vi "数据库查询.vi"() -> ()   [LabVIEW 2018]
uses:
  NPOI/net40/yt_ExcelLibrary.dll
  <vilib>/addons/database/Connection.llb/DB Tools Open Connec (String).vi
  <vilib>/addons/database/NI_Database_API.lvlib
  <vilib>/Utility/NIReport.llb/NI_report.lvclass
  <vilib>/addons/_office/NI_ReportGenerationToolkit.lvlib
  <vilib>/Utility/NIReport.llb/Excel/NI_Excel.lvclass
  <vilib>/addons/_office/_exclsub.llb/font.ctl
  <vilib>/ptbypt/NI_PtbyPt.lvlib
  FreeMem.dll
  <vilib>/addons/_office/excel.llb/Excel Easy Table (str).vi
panel:
  out "错误输出":errorcluster
  out "数字(0-1)":dbl
  out "Elapsed Time (s)":dbl caption="已用时间(s)"
  out "2天时间到释放资源":bool caption="结束"
  in  "Main Tab":enum32{""}(tab)
  in  "查询结果":i32(listbox)
  in  "时间范围OFF":bool
  out "查询状态":string
  in  "总成码OFF":bool
  in  "总成码":string
  in  "导出":bool
  in  "退出":bool
  in  "查询":bool
  in  "另存为":bool
  in  "二维码OFF":bool
  in  "二维码":string
  in  "结束日期":timestamp
  in  "起始日期":timestamp
  in  "数据类型":u16(ring) items=["ALL", "Online", "Offline", "Rework", "70站"]
  in  "产品状态":u16(ring) items=["ALL", "OK", "NG"]
  # "历史数据查询"
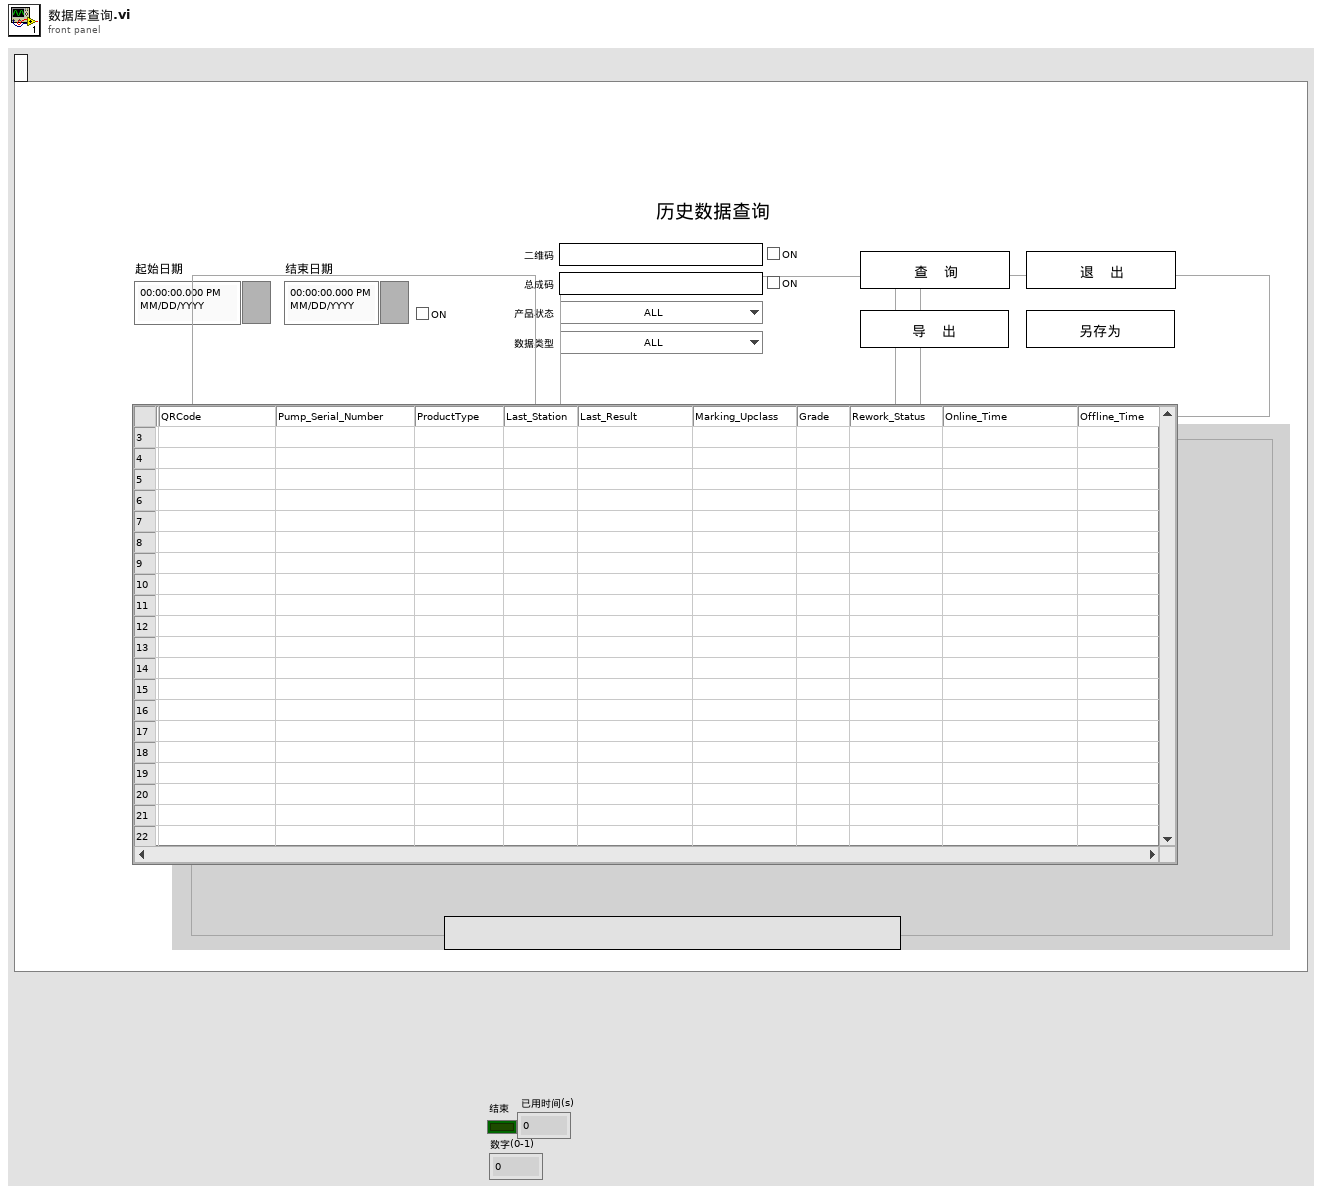
[diagram p1: front panel]
types:
  T1 = typedef "NI_ReportGenerationToolkit.lvlib/font.ctl" = cluster{"font name":string, "font size":dbl, "bold":u16, "italic":u16, "underline":u16, "strike through":u16, "font color":u32}
  T2 = enum16{"Standard Report", "HTML", "Word", "Excel"}
  T3 = enum16{"maximized", "minimized", "normal", "no change"}
  T4 = enum32{"Invalid", "Standard", "Closed", "Hidden", "Minimized", "Maximized"}
  T5 = typedef "NI_Database_API.lvlib/Conn ObjectReference.ctl" = refnum<k1>
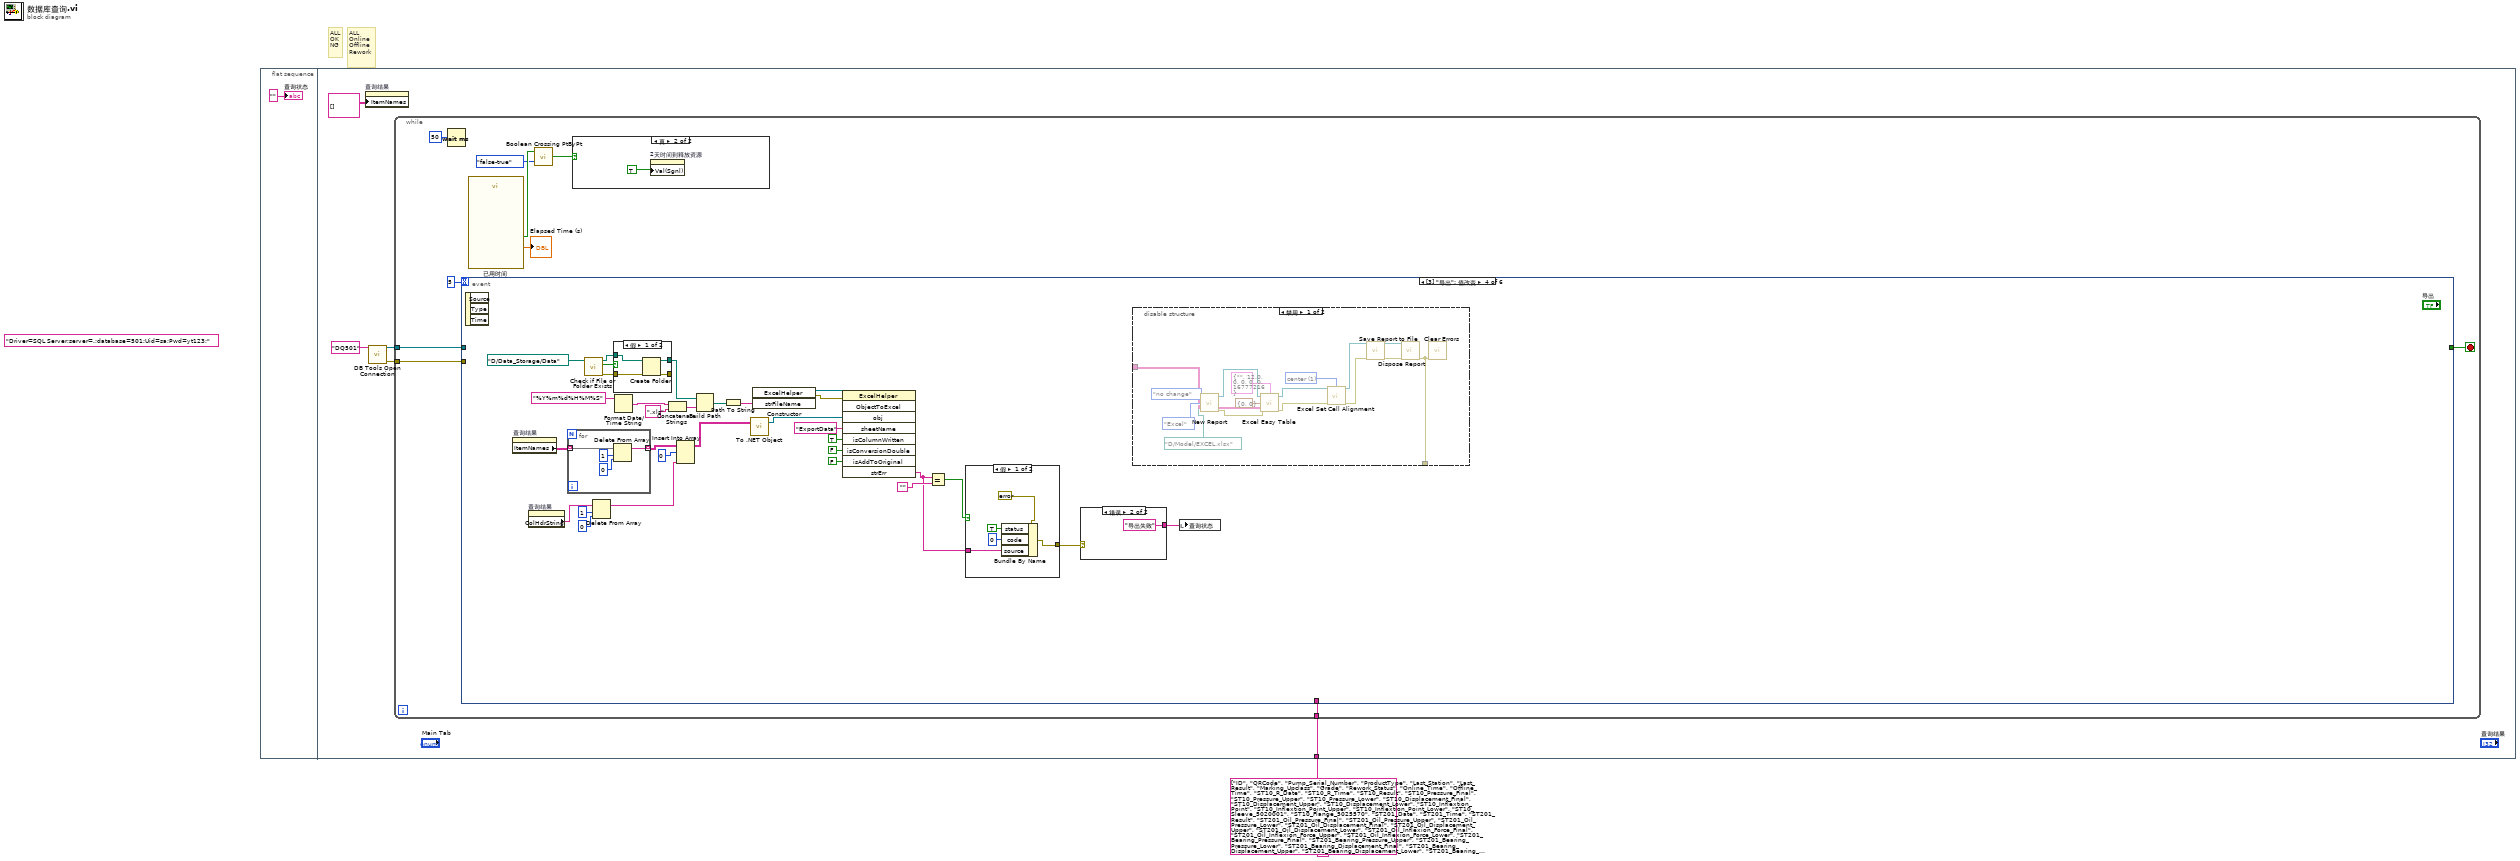
[diagram p0: block diagram]
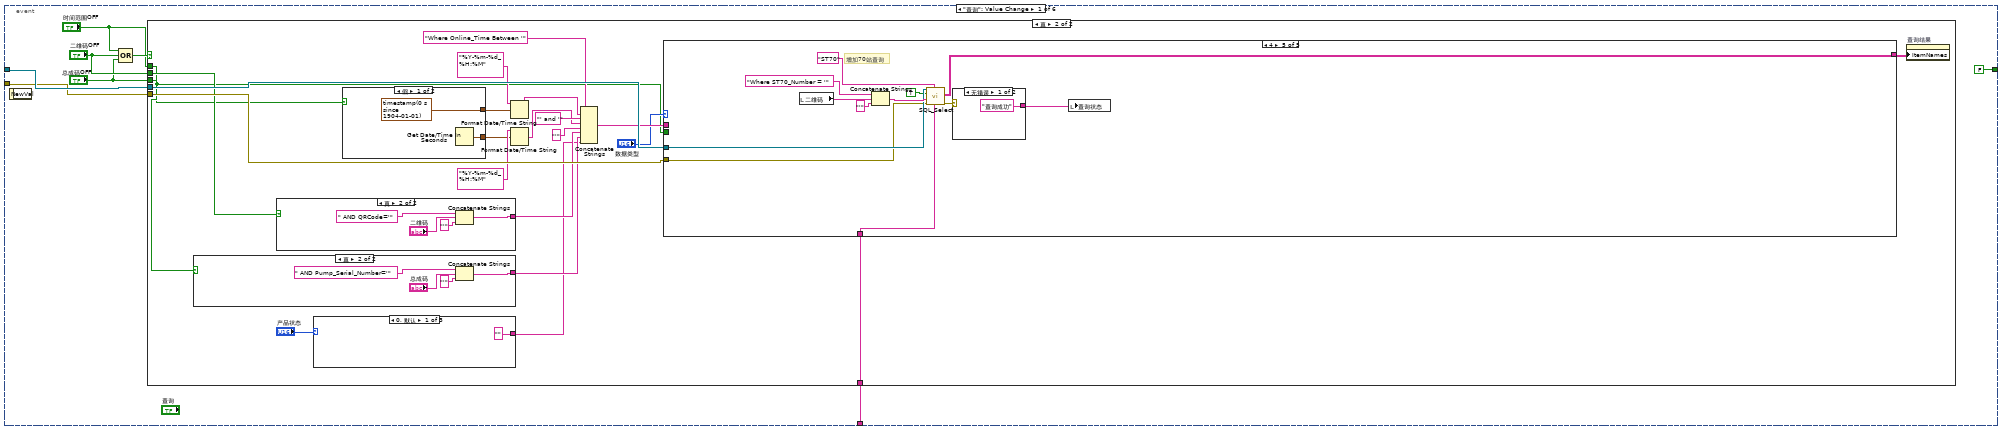
[diagram p3: hidden frame]
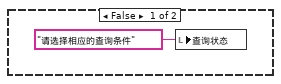
[diagram p4: hidden frame]
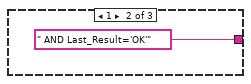
[diagram p5: hidden frame]
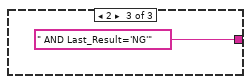
[diagram p6: hidden frame]
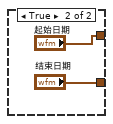
[diagram p7: hidden frame]
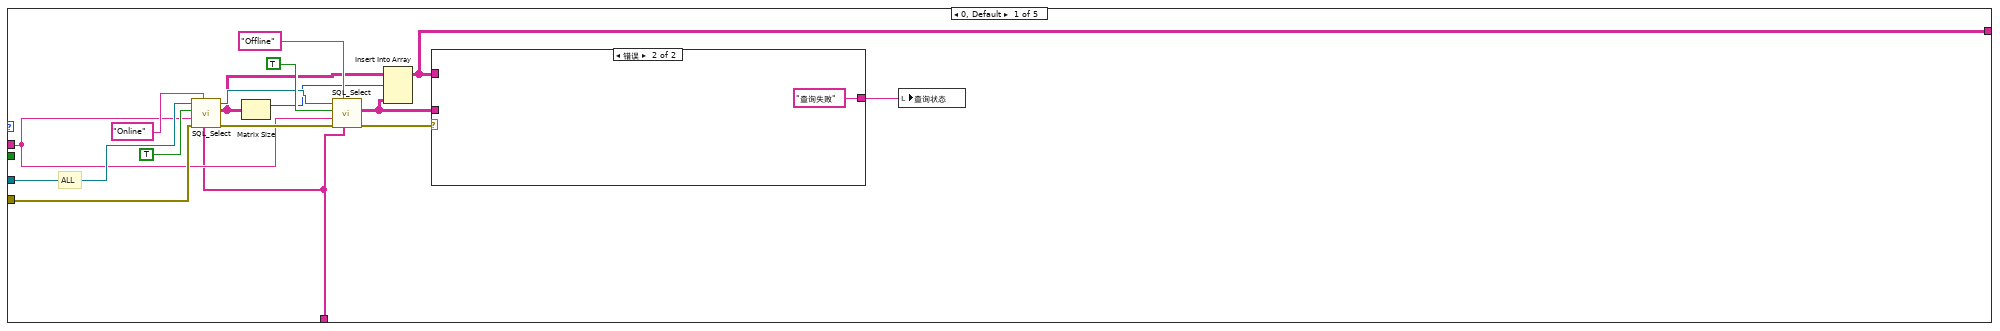
[diagram p8: hidden frame]
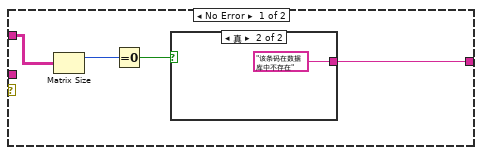
[diagram p9: hidden frame]
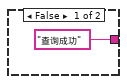
[diagram p10: hidden frame]
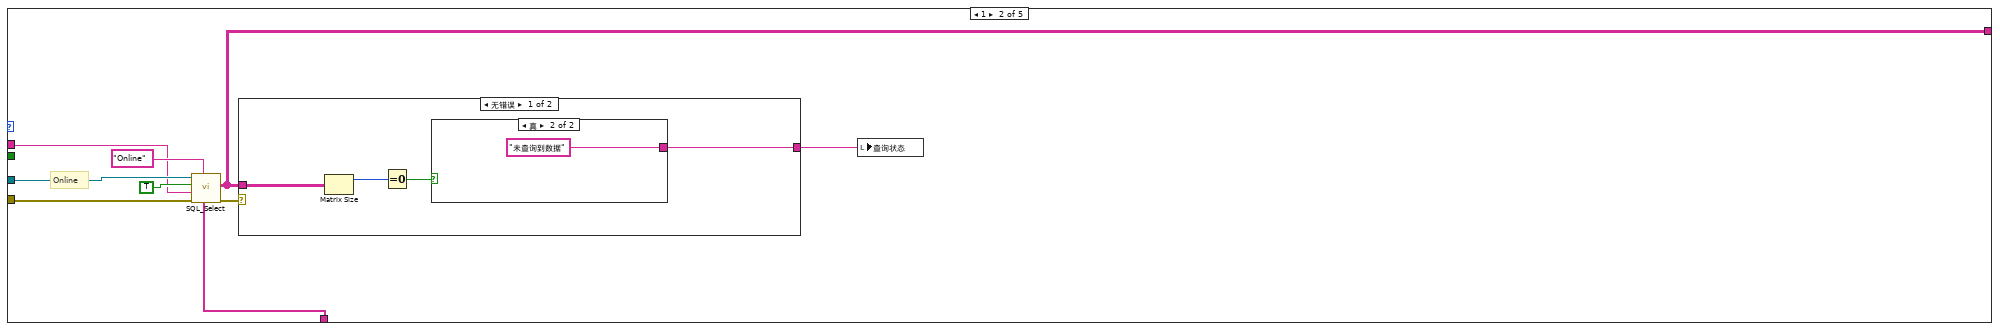
[diagram p11: hidden frame]
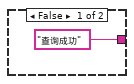
[diagram p12: hidden frame]
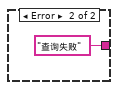
[diagram p13: hidden frame]
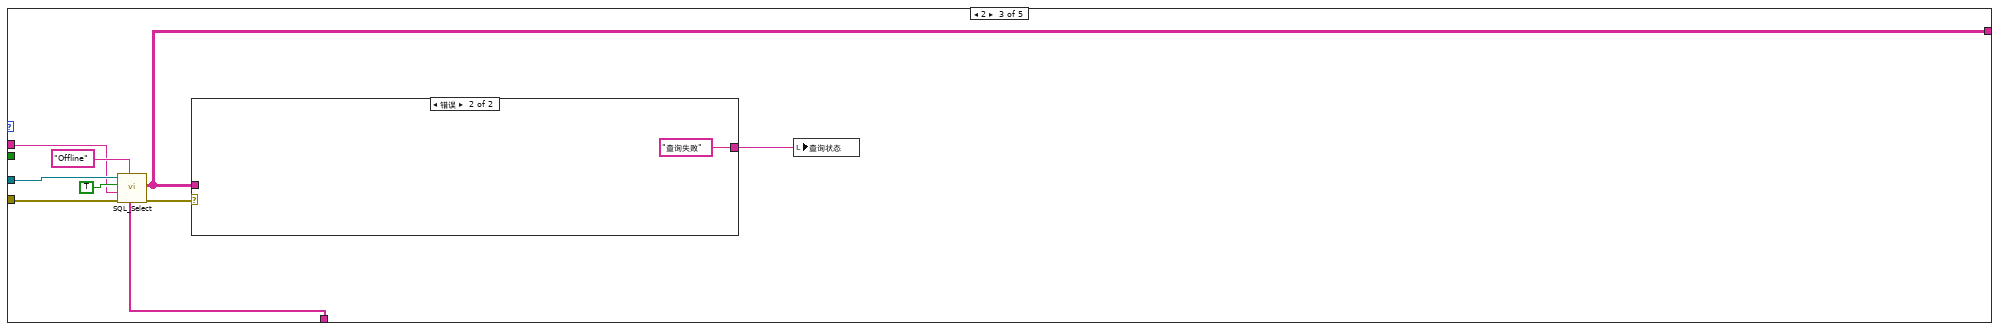
[diagram p14: hidden frame]
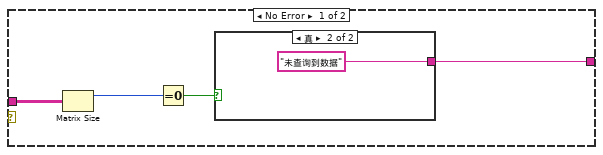
[diagram p15: hidden frame]
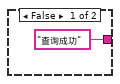
[diagram p16: hidden frame]
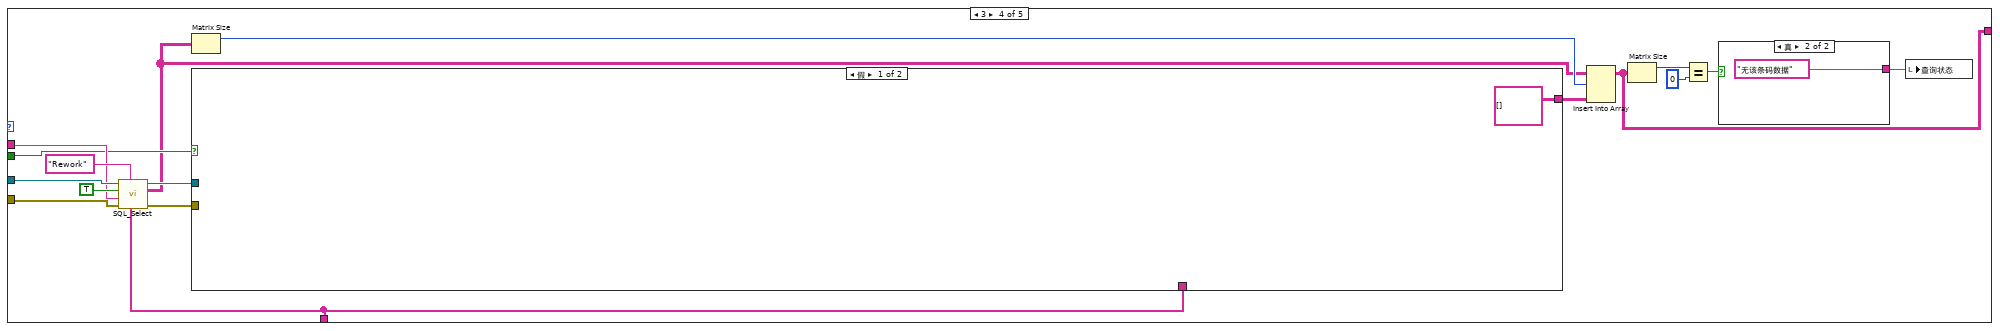
[diagram p17: hidden frame]
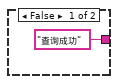
[diagram p18: hidden frame]
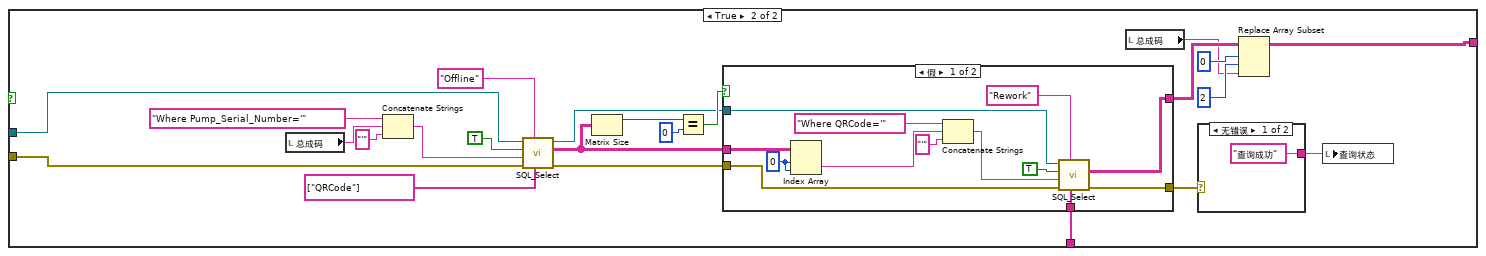
[diagram p19: hidden frame]
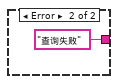
[diagram p20: hidden frame]
diagram:
  (unwired) "Driver=SQL Server;server=.;database=501;Uid=sa;Pwd=yt123;"
  # "ALL\nOK\nNG"
  # "ALL\nOnline\nOffline\nRework"
  n1 = flat-sequence {
    tunnel: string[] ["ID", "QRCode", "Pump_Serial_Number", "ProductType", "Last_Station", "Last_Result", "Marking_Upclass", "Grade", "Rework_Status", "Online_Time", "Offline_Time", "ST10_R_Date", "ST10_R_Time", "ST10_Result", "ST10_Pressure_Final", "ST10_Pressure_Upper", "ST10_Pressure_Lower", "ST10_Displacement_Final", "ST10_Displacement_Upper", "ST10_Displacement_Lower", "ST10_Inflextion_Point", "ST10_Inflextion_Point_Upper", "ST10_Inflextion_Point_Lower", "ST10_Sleeve_5020001", "ST10_Flange_5025570", "ST201_Date", "ST201_Time", "ST201_Result", "ST201_Oil_Pressure_Final", "ST201_Oil_Pressure_Upper", "ST201_Oil_Pressure_Lower", "ST201_Oil_Displacement_Final", "ST201_Oil_Displacement_Upper", "ST201_Oil_Displacement_Lower", "ST201_Oil_Inflexion_Force_Final", "ST201_Oil_Inflexion_Force_Upper", "ST201_Oil_Inflexion_Force_Lower", "ST201_Bearing_Pressure_Final", "ST201_Bearing_Pressure_Upper", "ST201_Bearing_Pressure_Lower", "ST201_Bearing_Displacement_Final", "ST201_Bearing_Displacement_Upper", "ST201_Bearing_Displacement_Lower", "ST201_Bearing_Inflexion_Force_Final", "ST201_Bearing_Inflexion_Force_Upper", "ST201_Bearing_Inflexion_Force_Lower", "ST202_Date", "ST202_Time", "ST202_Result", "ST202_Pressure_Final", "ST202_Pressure_Upper", "ST202_Pressure_Lower", "ST202_Displacement_Final", "ST202_Displacement_Upper", "ST202_Displacement_Lower", "ST202_Sealing_5026269", "ST202_Flange_5025570", "ST202_Shaft_5020526", "ST202_Ring_5020571", "ST202_Needle_bearing_5020570", "ST301_Date", "ST301_Time", "ST301_Result", "ST301_Shield", "ST301_Magnetic_flux_Left", "ST301_Magnetic_flux_Right", "ST301_Magnetic_flux_Upper", "ST301_Magnetic_flux_Lower", "ST301_PanelNumber", "ST302_Date", "ST302_Time", "ST302_Result", "ST302_PanelNumber", "ST303_Date", "ST303_Time", "ST303_Result", "ST303_PanelNumber", "ST303_Cam_ring_5020689", "ST303_Pin_5026280", "ST303_Rotor_5018111", "ST401_Date", "ST401_Time", "ST401_Result", "ST401_Shield", "ST401_PanelNumber", "ST402_Date", "ST402_Time", "ST402_Result", "ST402_Shield", "ST402_PanelNumber", "ST501_Date", "ST501_Time", "ST501_Result", "ST501_Shield", "ST501_PanelNumber", "ST502_Date", "ST502_Time", "ST502_Result", "ST502_PanelNumber", "ST502_Pressure_Final1", "ST502_Pressure_Upper1", "ST502_Pressure_Lower1", "ST502_Distance_Final1", "ST502_Distance_Upper1", "ST502_Distance_Lower1", "ST502_Pressure_Final2", "ST502_Pressure_Upper2", "ST502_Pressure_Lower2", "ST502_Distance_Final2", "ST502_Distance_Upper2", "ST502_Distance_Lower2", "ST502_Inflexion_force_Left_Final", "ST502_Inflexion_force_Left_Upper", "ST502_Inflexion_force_Left_Lower", "ST502_Inflexion_force_Right_Final", "ST502_Inflexion_force_Right_Upper", "ST502_Inflexion_force_Right_Lower", "ST503_Date", "ST503_Time", "ST503_Result", "ST503_PanelNumber", "ST503_Pin", "ST503_Position_degree", "ST504_Date", "ST504_Time", "ST504_Result", "ST504_PanelNumber", "ST504_Small_Sealing_Ring_Exit", "ST504_Small_Sealing_Ring_Excess", "ST504_Big_Sealing_Ring_Exit", "ST504_Big_Sealing_Ring_Number", "ST504_Retaining_Ring_LH2110811", "ST504_Pressure_Plate_5020472", "ST504_O_ring_5003059", "ST504_O_ring_5003061", "ST504_Spring_Dowel_Pin_5018182", "ST601_Date", "ST601_Time", "ST601_Result", "ST601_PanelNumber", "ST602_Date", "ST602_Time", "ST602_Result", "ST602_PanelNumber", "ST603_Date", "ST603_Time", "ST603_Result", "ST603_PanelNumber", "ST603_Spring_Retainer_5020834", "ST603_Spring_5024602", "ST603_Retaining_ring_5018568", "ST603_Disc_spring_5005082", "ST603_Bushing_5024673", "ST70_Number", "ST70_Date", "ST70_Time", "ST70_Result", "ST70_Pressure_Final1", "ST70_Pressure_Upper1", "ST70_Pressure_Lower1", "ST70_Distance_Final1", "ST70_Distance_Upper1", "ST70_Distance_Lower1", "ST70_Pressure_Final2", "ST70_Pressure_Upper2", "ST70_Pressure_Lower2", "ST70_Distance_Final2", "ST70_Distance_Upper2", "ST70_Distance_Lower2", "ST70_Inflexion_force_Left_Final", "ST70_Inflexion_force_Left_Upper", "ST70_Inflexion_force_Left_Lower", "ST70_Inflexion_force_Right_Final", "ST70_Inflexion_force_Right_Upper", "ST70_Inflexion_force_Right_Lower", "ST70_Housing_5025351", "ST70_Bushing_5025400", "ST80_Date", "ST80_Time", "ST80_Result", "ST80_Flat_Sael_5020064", "ST80_Spring_5024883", "ST80_Spring_Plate_5025473", "ST901_Date", "ST901_Time", "ST901_Result", "ST901_Torque1", "ST901_Angle1", "ST901_Gradient1", "ST901_Torque2", "ST901_Angle2", "ST901_Gradient2", "ST901_Torque3", "ST901_Angle3", "ST901_Gradient3", "ST901_Torque4", "ST901_Angle4", "ST901_Gradient4", "ST901_Torque5", "ST901_Angle5", "ST901_Gradient5", "ST901_Torque_Upper", "ST901_Torque_Lower", "ST901_Angle_Upper", "ST901_Angle_Lower", "ST901_Gradient_Upper", "ST901_Gradient_Lower", "ST902_Date", "ST902_Time", "ST902_Result", "ST902_Leakage1", "ST902_Leakage2", "ST902_Leakage3", "ST902_Leakage_Upper", "ST902_Leakage_Lower"] ("要读取的列名") -> [w4]
    frame #0 {
      "查询状态" <- "" ("查询状态")
    }
    frame #1 {
      n2 = property on="查询结果" class="MCListbox (严格)"("ItemNames"=string[][] [] ("项名")) -> ()  [unwired: 2 in, 2 out]
      n3 = call-poly <vilib>:"DB Tools Open Connection.vi"("connection information"="DQ501") -> ("error out"=w6:errorcluster, "connection reference"=w7:T5)  [unwired: 7 in]
      n4 = while {
        tunnel: w7 -> [w17]
        tunnel: w6 -> [w16]
        tunnel: w4 -> [w8]
        stop <- w15 stop-if-true
        n5 = Wait (ms)(milliseconds to wait=u32 50 ("等待时间（毫秒）")) -> ()  [unwired: 1 out]
        n6 = event shown="[3] \"导出\": 值改变" {
          selector: _ -> [_ _ _ _ _ _]
          dyn-events: _ -> [_ _ _ _ _ _]
          timeout: 5 -> [_ _ _ _ _ _]
          tunnel: w17 -> [w26 _ _ _ w279 _]
          tunnel: w16 -> [w25 _ _ _ w278 _]
          tunnel: [FALSE ("NewVal") _ FALSE ("NewVal") _ w280 _] -> w15
          tunnel: w8 -> [w19 _ _ _ _ _]
          event "查询": Value Change {
            n7 = event-data() -> ()  [unwired: 1 in, 1 out]
            n8 = Compound Arithmetic op=OR("时间范围OFF", "二维码OFF", "总成码OFF") -> (w21:bool)
            n9 = case shown="真" w21 {
              tunnel: w26 -> [_ w49]
              tunnel: w25 -> [_ w48]
              tunnel: "二维码OFF" -> [_ w34]
              tunnel: "总成码OFF" -> [_ w33]
              tunnel: "时间范围OFF" -> [_ w32]
              tunnel: w19 -> [_ w28]
              frame False {
                n10 = local write "查询状态"("请选择相应的查询条件" ("查询状态")) -> ()
              }
              frame True {
                n11 = case shown="真" w33 {
                  tunnel: ["" w188] -> w36
                  frame False {
                  }
                  frame True {
                    n12 = Concatenate Strings(" AND Pump_Serial_Number='" ("字符串"), "总成码", "'" ("字符串")) -> (w188:string)
                  }
                }
                n13 = case shown="真" w34 {
                  tunnel: ["" w192] -> w39
                  frame False {
                  }
                  frame True {
                    n14 = Concatenate Strings(" AND QRCode='" ("字符串"), "二维码", "'" ("字符串")) -> (w192:string)
                  }
                }
                n15 = case shown="0, 默认" "产品状态" {
                  tunnel: ["" " AND Last_Result='OK'" ("字符串") " AND Last_Result='NG'" ("字符串")] -> w30
                  frame 0, Default {
                  }
                  frame 1 {
                  }
                  frame 2 {
                  }
                }
                n16 = case shown="假" w32 {
                  tunnel: [timestamp(0 s since 1904-01-01) ("起始日期") "起始日期"] -> w44
                  tunnel: [w53 "结束日期"] -> w41
                  frame False {
                    n17 = Get Date/Time In Seconds() -> (seconds since 1Jan1904=w53:timestamp)
                  }
                  frame True {
                  }
                }
                n18 = Format Date/Time String(time format string (%c)="%Y-%m-%d_%H:%M" ("时间格式字符串(%c)"), seconds (now)=w44) -> (date/time string=w43:string)  [unwired: 1 in]
                n19 = Format Date/Time String(time format string (%c)="%Y-%m-%d_%H:%M" ("时间格式字符串(%c)"), seconds (now)=w41) -> (date/time string=w40:string)  [unwired: 1 in]
                n20 = Concatenate Strings("Where Online_Time Between '" ("查询语句"), w43, "' and '" ("字符串"), w40, "'" ("字符串"), w39, w36, w30) -> (w38:string)
                n21 = case shown="4" "数据类型" {
                  tunnel: w49 -> [w72 w84 w100 w126 w179]
                  tunnel: w48 -> [w71 w83 w99 w125 w176]
                  tunnel: w38 -> [w62 w82 w98 w124 _]
                  tunnel: [w58 w81 w97 w117 w174] -> w29
                  tunnel: w33 -> [_ _ _ w123 _]
                  tunnel: w28 -> [w57 w80 w96 w112 w172]
                  frame 0, Default {
                    # "ALL"
                    n22 = call "SQL_Select.vi"("要读取的列名"=w57, "表名"="Online", "error in (no error)"=w71, "查询语句"=w62, "查询条件"=TRUE, "connection reference"=w72) -> ("error out"=w67:errorcluster, "数据"=w64:string[][], "connection reference out"=w66:T5)  [unwired: 3 in]
                    n23 = Matrix Size(0:w64) -> (1:w63:i32)  [unwired: 1 out]
                    n24 = call "SQL_Select.vi"("要读取的列名"=w57, "表名"="Offline", "error in (no error)"=w67, "查询语句"=w62, "查询条件"=TRUE, "connection reference"=w66) -> ("error out"=w61:errorcluster, "数据"=w59:string[][])  [unwired: 3 in, 1 out]
                    n25 = Insert Into Array(array=w64, index (row)=w63, new element=w59) -> (w58:string[][])  [unwired: 1 in]
                    n26 = case shown="错误" w61 {
                      tunnel: [w74 "查询失败"] -> w60
                      tunnel: w59 -> [_ _]
                      tunnel: w58 -> [w73 _]
                      frame No Error {
                        n27 = Matrix Size(0:w73) -> (1:w76:i32)  [unwired: 1 out]
                        n28 = Equal To 0?(x=w76) -> (x = 0?=w75:bool)
                        n29 = case shown="真" w75 {
                          tunnel: ["查询成功" "该条码在数据库中不存在"] -> w74
                          frame False {
                          }
                          frame True {
                          }
                        }
                      }
                      frame Error {
                      }
                    }
                    n30 = local write "查询状态"(w60) -> ()
                  }
                  frame 1 {
                    # "Online"
                    n31 = call "SQL_Select.vi"("要读取的列名"=w80, "表名"="Online", "error in (no error)"=w83, "查询语句"=w82, "查询条件"=TRUE, "connection reference"=w84) -> ("error out"=w86:errorcluster, "数据"=w81:string[][])  [unwired: 3 in, 1 out]
                    n32 = case shown="无错误" w86 {
                      tunnel: [w90 "查询失败"] -> w85
                      tunnel: w81 -> [w89 _]
                      frame No Error {
                        n33 = Matrix Size(0:w89) -> (1:w92:i32)  [unwired: 1 out]
                        n34 = Equal To 0?(x=w92) -> (x = 0?=w91:bool)
                        n35 = case shown="真" w91 {
                          tunnel: ["查询成功" "未查询到数据"] -> w90
                          frame False {
                          }
                          frame True {
                          }
                        }
                      }
                      frame Error {
                      }
                    }
                    n36 = local write "查询状态"(w85) -> ()
                  }
                  frame 2 {
                    n37 = call "SQL_Select.vi"("要读取的列名"=w96, "表名"="Offline", "error in (no error)"=w99, "查询语句"=w98, "查询条件"=TRUE, "connection reference"=w100) -> ("error out"=w102:errorcluster, "数据"=w97:string[][])  [unwired: 3 in, 1 out]
                    n38 = case shown="错误" w102 {
                      tunnel: [w106 "查询失败"] -> w101
                      tunnel: w97 -> [w105 _]
                      frame No Error {
                        n39 = Matrix Size(0:w105) -> (1:w108:i32)  [unwired: 1 out]
                        n40 = Equal To 0?(x=w108) -> (x = 0?=w107:bool)
                        n41 = case shown="真" w107 {
                          tunnel: ["查询成功" "未查询到数据"] -> w106
                          frame False {
                          }
                          frame True {
                          }
                        }
                      }
                      frame Error {
                      }
                    }
                    n42 = local write "查询状态"(w101) -> ()
                  }
                  frame 3 {
                    n43 = call "SQL_Select.vi"("要读取的列名"=w112, "表名"="Rework", "error in (no error)"=w125, "查询语句"=w124, "查询条件"=TRUE, "connection reference"=w126) -> ("error out"=w122:errorcluster, "数据"=w119:string[][], "connection reference out"=w121:T5)  [unwired: 3 in]
                    n44 = Matrix Size(0:w119) -> (1:w120:i32)  [unwired: 1 out]
                    n45 = case shown="假" w123 {
                      tunnel: w122 -> [_ w154]
                      tunnel: w121 -> [_ w153]
                      tunnel: [string[][] [] ("数据") w133] -> w118
                      tunnel: w112 -> [_ w132]
                      frame False {
                      }
                      frame True {
                        n46 = local read "总成码"() -> (w148:string)
                        n47 = Concatenate Strings("Where Pump_Serial_Number='" ("查询语句"), w148, "'" ("字符串")) -> (w147:string)
                        n48 = call "SQL_Select.vi"("要读取的列名"=string[] ["QRCode"], "表名"="Offline", "error in (no error)"=w154, "查询语句"=w147, "查询条件"=TRUE, "connection reference"=w153) -> ("error out"=w141:errorcluster, "数据"=w140:string[][], "connection reference out"=w142:T5)  [unwired: 3 in]
                        n49 = Matrix Size(0:w140) -> (1:w145:i32)  [unwired: 1 out]
                        n50 = Equal?(x=w145, y=0) -> (x = y?=w143:bool)
                        n51 = case shown="假" w143 {
                          tunnel: w142 -> [w169 _]
                          tunnel: w141 -> [w168 w171]
                          tunnel: [w165 string[][] [] ("数据")] -> w137
                          tunnel: [w164 w171] -> w138
                          tunnel: w140 -> [w161 _]
                          tunnel: w132 -> [w157 _]
                          frame False {
                            w160 = 0 ("索引 (行)")
                            n52 = Index Array(array=w161, index (row)=w160, index (col)=w160) -> (element=w159:string)
                            n53 = Concatenate Strings("Where QRCode='" ("查询语句"), w159, "'" ("字符串")) -> (w163:string)
                            n54 = call "SQL_Select.vi"("要读取的列名"=w157, "表名"="Rework", "error in (no error)"=w168, "查询语句"=w163, "查询条件"=TRUE, "connection reference"=w169) -> ("error out"=w164:errorcluster, "数据"=w165:string[][])  [unwired: 3 in, 1 out]
                          }
                          frame True {
                          }
                        }
                        n55 = local read "总成码"() -> (w134:string)
                        n56 = case shown="无错误" w138 {
                          tunnel: ["查询成功" "查询失败"] -> w139
                          frame No Error {
                          }
                          frame Error {
                          }
                        }
                        n57 = Replace Array Subset(array=w137, new element=w134, index (row)=0 ("索引 (行)"), index (col)=2 ("禁用的索引 (列)")) -> (w133:string[][])
                        n58 = local write "查询状态"(w139) -> ()
                      }
                    }
                    n59 = Insert Into Array(array=w119, index (row)=w120, new element=w118) -> (w117:string[][])  [unwired: 1 in]
                    n60 = Matrix Size(0:w117) -> (1:w116:i32)  [unwired: 1 out]
                    n61 = Equal?(x=w116, y=0) -> (x = y?=w113:bool)
                    n62 = case shown="真" w113 {
                      tunnel: ["查询成功" "无该条码数据"] -> w114
                      frame False {
                      }
                      frame True {
                      }
                    }
                    n63 = local write "查询状态"(w114) -> ()
                  }
                  frame 4 {
                    # "增加70站查询"
                    n64 = local read "二维码"() -> (w182:string)
                    n65 = Concatenate Strings("Where ST70_Number = '" ("查询语句"), w182, "'" ("字符串")) -> (w180:string)
                    n66 = call "SQL_Select.vi"("要读取的列名"=w172, "表名"="ST70", "error in (no error)"=w176, "查询语句"=w180, "查询条件"=TRUE, "connection reference"=w179) -> ("error out"=w175:errorcluster, "数据"=w174:string[][])  [unwired: 3 in, 1 out]
                    n67 = case shown="无错误" w175 {
                      tunnel: ["查询成功" "查询失败"] -> w173
                      frame No Error {
                      }
                      frame Error {
                      }
                    }
                    n68 = local write "查询状态"(w173) -> ()
                  }
                }
                n69 = property on="查询结果" class="MCListbox (严格)"("ItemNames"=w29) -> ()  [unwired: 2 in, 2 out]
              }
            }
          }
          event Timeout {
            n70 = event-data() -> ()  [unwired: 1 in, 3 out]
          }
          event "另存为": Value Change {
            n71 = event-data() -> ()  [unwired: 1 in, 1 out]
            n72 = property on="查询结果" class="MCListbox (严格)"() -> ("ItemNames"=w197:string[][])  [unwired: 2 in, 2 out]
            n73 = for {
              tunnel: w197 -> [w209] mode=indexing
              tunnel: [w206] -> w201 mode=indexing
              n74 = Delete From Array(array=w209, length=1 ("长度"), index=0 ("索引")) -> (array with subset deleted=w206:string[])  [unwired: 1 out]
            }
            n75 = property on="查询结果" class="MCListbox (严格)"() -> ("ColHdrString"=w196:string[])  [unwired: 2 in, 2 out]
            n76 = Delete From Array(array=w196, length=1 ("长度"), index=0 ("索引")) -> (array with subset deleted=w200:string[])  [unwired: 1 out]
            n77 = Insert Into Array(array=w201, index (row)=0 ("索引"), new element=w200) -> (w199:string[][])  [unwired: 1 in]
            n78 = call "Save to EXCEL.vi"("text data"=w199) -> ("error out"=w198:errorcluster)  [unwired: 10 in]
            n79 = call <vilib>:"Clear Errors.vi"("error in (no error)"=w198) -> ()  [unwired: 5 in, 2 out]
          }
          event "导出": Value Change {
            n80 = event-data() -> ()  [unwired: 1 in, 3 out]
            n81 = property on="查询结果" class="MCListbox (严格)"() -> ("ItemNames"=w225:string[][])  [unwired: 2 in, 2 out]
            n82 = property on="查询结果" class="MCListbox (严格)"() -> ("ColHdrString"=w224:string[])  [unwired: 2 in, 2 out]
            n83 = for {
              tunnel: w225 -> [w275] mode=indexing
              tunnel: [w272] -> w237 mode=indexing
              n84 = Delete From Array(array=w275, length=1 ("长度"), index=0 ("索引")) -> (array with subset deleted=w272:string[])  [unwired: 1 out]
            }
            n85 = call <vilib>:"Check if File or Folder Exists.vi"("path"=path "D:/Data_Storage/Data" ("文件路径（使用对话框）")) -> ("error out"=w232:errorcluster, "file or folder exists?"=w234:bool, "dup path"=w233:path)  [unwired: 8 in]
            n86 = Delete From Array(array=w224, length=1 ("长度"), index=0 ("索引")) -> (array with subset deleted=w236:string[])  [unwired: 1 out]
            n87 = case shown="假" w234 {
              tunnel: w233 -> [w269 w271]
              tunnel: [w268 w271] -> w228
              tunnel: w232 -> [w267 w270]
              tunnel: [w266 w270] -> _
              frame False {
                n88 = Create Folder(path (use dialog)=w269, error in=w267) -> (created path=w268:path, error out=w266:errorcluster)  [unwired: 1 in, 1 out]
              }
              frame True {
              }
            }
            n89 = Format Date/Time String(time format string (%c)="%Y%m%d%H%M%S" ("时间格式字符串(%c)")) -> (date/time string=w230:string)  [unwired: 2 in]
            n90 = Concatenate Strings(w230, ".xls" ("字符串")) -> (w227:string)
            n91 = Insert Into Array(array=w237, index (row)=0 ("索引"), new element=w236) -> (w219:string[][])  [unwired: 1 in]
            n92 = Build Path(base path=w228, name or relative path=w227) -> (appended path=w223:path)
            n93 = Path To String(path=w223) -> (string=w222:string)
            n94 = call <vilib>:"To .NET Object.vi"("anything"=w219) -> (".NET object"=w218:refnum<k24>)  [unwired: 1 in, 1 out]
            n95 = constructor class="ExcelHelper"("strFileName"=w222) -> (reference out=w221:refnum<k24>, error out=w220:errorcluster)  [unwired: 3 in, 2 out]
            n96 = invoke class="ExcelHelper" method="ObjectToExcel"(reference=w221, error in=w220, "obj"=w218, "sheetName"="ExportData", "isColumnWritten"=TRUE, "isConversionDouble"=FALSE, "isAddToOriginal"=FALSE) -> ("strErr"=w210:string)  [unwired: 2 in, 8 out]
            n97 = Equal?(x=w210, y="") -> (x = y?=w212:bool)
            n98 = case shown="假" w212 {
              tunnel: [w244 errorcluster {"status"=FALSE, "code"=0, "source"=""} ("error IO")] -> w211
              tunnel: w210 -> [w241 _]
              frame False {
                n99 = Bundle By Name(cluster=errorcluster {"status"=FALSE, "code"=0, "source"=""} ("error IO"), "status"=TRUE, "code"=0, "source"=w241) -> (w244:errorcluster)
              }
              frame True {
              }
            }
            n100 = case shown="错误" w211 {
              tunnel: ["导出成功" "导出失败"] -> w226
              frame No Error {
              }
              frame Error {
              }
            }
            n101 = disable-structure shown="禁用" {
              disable-tunnel: _ -> [w250 _]
              disable-tunnel: [w247 _] -> _
              frame Disabled {
                w260 = 1 items=["left", "center", "right"] ("horizontal alignment (left)")
                n102 = call <vilib>:"New Report.vi"("window state (normal)"=T3."no change", "report type"=T2."Excel", "template (empty)"=path "D:/Model/EXCEL.xlsx") -> ("report out"=w256:refnum<class "NI_report.lvclass">, "error out"=w257:errorcluster)  [unwired: 11 in]
                n103 = call-poly <vilib>:"Excel Easy Table.vi"("report in"=w256, "font"=T1 {"font name"="", "font size"=12.0, "bold"=0, "italic"=0, "underline"=0, "strike through"=0, "font color"=16777216}, "start (0, 0)"=cluster{"row":i32, "column":i32} {"row"=0, "column"=0}, "text data"=w250, "error in (no error)"=w257) -> ("report out"=w258:refnum<class "NI_report.lvclass">, "error out"=w259:errorcluster)  [unwired: 6 in, 3 out]
                n104 = call <vilib>:"Excel Set Cell Alignment.vi"("report in"=w258, "horizontal alignment (left)"=w260, "error in (no error)"=w259) -> ("report out"=w251:refnum<class "NI_report.lvclass">, "error out"=w254:errorcluster)  [unwired: 11 in]
                n105 = call-dynamic "Save Report to File.vi"("report in"=w251, "error in (no error)"=w254) -> ("report out"=w252:refnum<class "NI_report.lvclass">, "report file path"=w248:path, "error out"=w253:errorcluster)  [unwired: 11 in]
                n106 = call-dynamic "Dispose Report.vi"("report in"=w252, "error in (no error)"=w253) -> ("error out"=w247:errorcluster)  [unwired: 13 in]
                n107 = call <vilib>:"Clear Errors.vi"("error in (no error)"=w247) -> ()  [unwired: 5 in, 2 out]
              }
              frame Enabled {
              }
            }
            n108 = local write "查询状态"(w226) -> ()
          }
          event "退出": Value Change {
            n109 = event-data() -> ("NewVal"=w280:bool)  [unwired: 1 in]
            n110 = call <vilib>:"DB Tools Close Connection.vi"("error in (no error)"=w278, "connection reference"=w279) -> ()  [unwired: 5 in, 1 out]
            n111 = control-ref of="本VI"() -> (w277:refnum<vi>)
            n112 = property class="VI"(reference=w277, "FP.State"=T4."Closed" ("前面板窗口:状态")) -> ()  [unwired: 1 in, 2 out]
          }
          event "2天时间到释放资源": Value Change {
            n113 = event-data() -> ()  [unwired: 1 in, 3 out]
            n114 = dll-call lib="PTH2¡abs E$èå·åæ³°ç§æè¡ä»½æéå¬å¸é¡¹ç®éº¦æ ¼çº³ç¨åºDQ381DQ501æ¹é -YT20-0315011-501ç¨åº 2018ç-20210909501-1ProjectFreeMem.dll" fn="FreeMem"() -> (error out=→"错误输出":errorcluster)  [unwired: 4 in, 1 out]
            n115 = Random Number (0-1)() -> (number: 0 to 1=→"数字(0-1)":dbl)
          }
        }
        n116 = call "已用时间"() -> ("Elapsed Time (s)"=→"Elapsed Time (s)":dbl, "Time has Elapsed"=w11:bool)  [unwired: 12 in, 6 out]
        n117 = call <vilib>:"Boolean Crossing PtByPt.vi"("direction"=enum16{"either", "false-true", "true-false"}."false-true", "input"=w11) -> ("crossing"=w10:bool)  [unwired: 1 in]
        n118 = case shown="真" w10 {
          frame False {
          }
          frame True {
            n119 = property on="2天时间到释放资源" class="Bool (严格)"("Val(Sgnl)"=TRUE ("值(信号)")) -> ()  [unwired: 2 in, 2 out]
          }
        }
      }
    }
  }
